vi "PromVIEW Instantiate WS.vi"(8 "error in (no error)":errorcluster, 9 "Web Resources Base Path":path, 10 "Web Service Name":string, 11 "Project Reference":refnum<vi>) -> (0 "Error Out":errorcluster)   [LabVIEW 2020]
uses:
  <resource>/Framework/Providers/ws_project_provider/common/Web Service VI Type.ctl
  <resource>/Framework/Providers/ws_project_provider/common/Web Service VI Method.ctl
  <resource>/Framework/Providers/ws_project_provider/common/Web Service VI Output Type.ctl
  <resource>/Framework/Providers/ws_project_provider/common/Web Service VI Output Format.ctl
  <resource>/Framework/Providers/ws_project_provider/common/NI Web Service Provider.lvlib
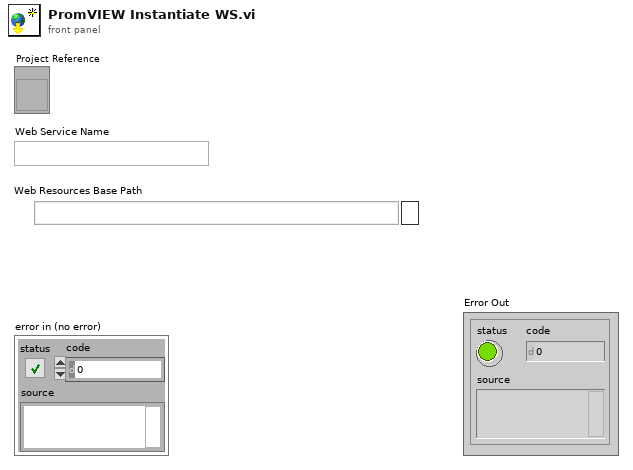
[diagram p1: front panel]
types:
  T1 = typedef "NI Web Service Provider.lvlib/Web Service VI Output Format.ctl" = enum16{"<DUMMY>", "Text", "XML", "HTML", "JSON"}
  T2 = typedef "NI Web Service Provider.lvlib/Web Service VI Output Type.ctl" = enum16{"Terminal", "Stream"}
  T3 = typedef "NI Web Service Provider.lvlib/Web Service VI Method.ctl" = enum16{"<DUMMY>", "GET", "PUT", "POST", "DELETE", "OPTIONS", "HEAD", "TRACE"}
  T4 = typedef "NI Web Service Provider.lvlib/Web Service VI Type.ctl" = enum16{"<DUMMY>", "Web Method", "Auxiliary", "Internal", "Content"}
  T5 = cluster{"Item URL":string, "Item ID":string, "Item Index":i32, "Specific Type":string}
  T6 = typedef "ItemRef.ctl" = u64
  T7 = typedef "NI Web Service Provider.lvlib/Web Service VI.ctl" = cluster{"item":u64, "item ID":string, "Web Service VI Type":T4, "Method":T3, "Load at startup":bool, "Keep in memory":bool, "Output type":T2, "Output format":T1, "Use headers":bool, "Buffered":bool, "Require API key":bool, "Permissions":string, "Standard URL":bool, "Include VI name in URL":bool, "Custom URL":string, "Required Privilege":string}
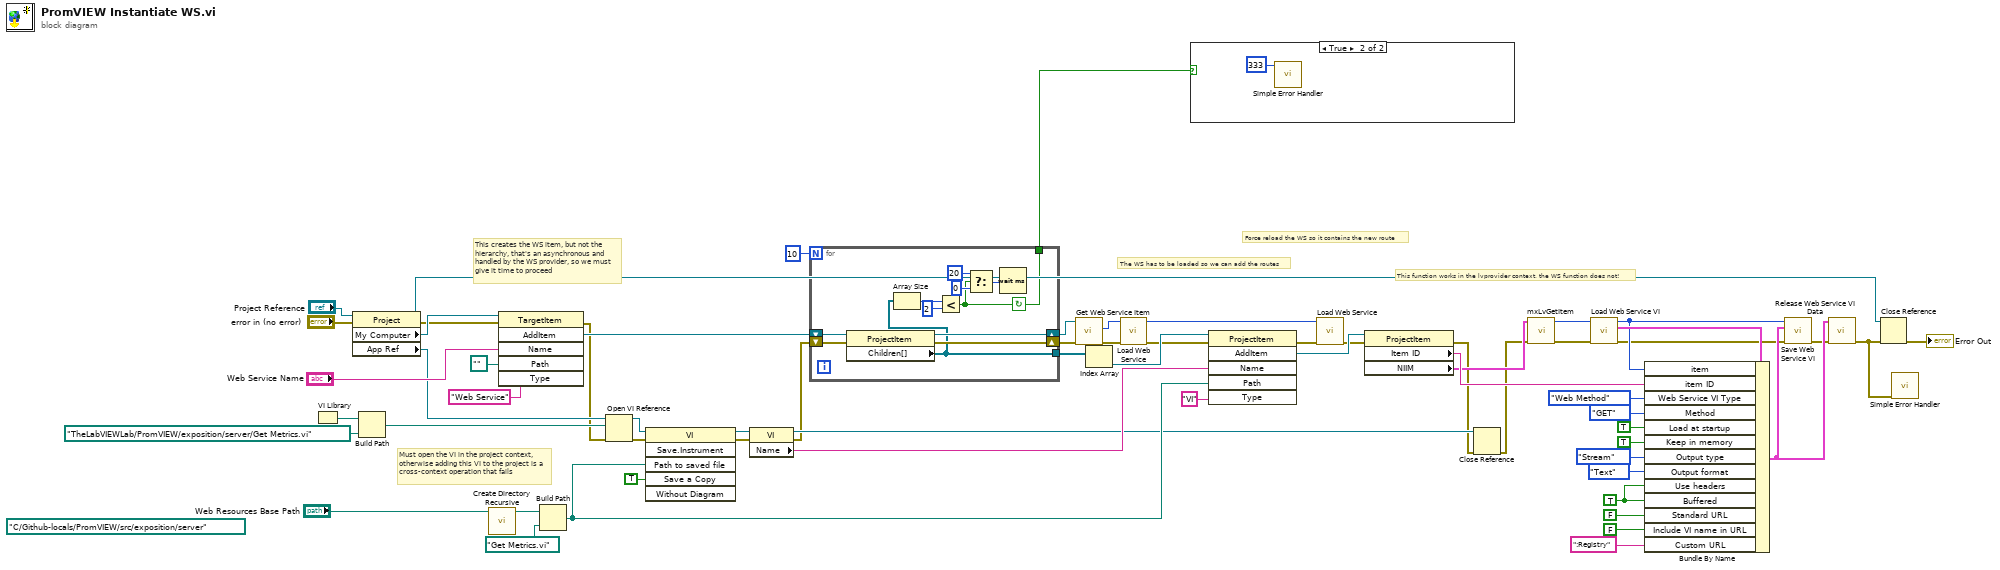
[diagram p0: block diagram]
diagram:
  w16 = TRUE ("Use headers")
  (unwired) path "C:/Github-locals/PromVIEW/src/exposition/server" ("name or relative path")
  # "Force reload the WS so it contains the new route"
  # "The WS has to be loaded so we can add the routes"
  # "This creates the WS item, but not the hierarchy, that's an asynchronous and handled by the WS provider, so we must give it time to proceed"
  # "This function works in the lvprovider context, the WS function does not!"
  # "Must open the VI in the project context, otherwise adding this VI to the project is a cross-context operation that fails"
  n1 = VI Library() -> (path=w49:path)
  n2 = property class="Project"(reference="Project Reference", error in="error in (no error)") -> (reference out=w50:refnum<vi>, error out=w56:errorcluster, "My Computer"=w62:refnum<vi>, "App Ref"=w41:refnum<vi>)
  n3 = Build Path(base path=w49, name or relative path=path "TheLabVIEWLab/PromVIEW/exposition/server/Get Metrics.vi") -> (appended path=w42:path)
  n4 = call <vilib>:"Create Directory Recursive.vi"("directory"="Web Resources Base Path") -> ("directory copy"=w58:path)  [unwired: 4 in, 2 out]
  n5 = invoke class="TargetItem" method="AddItem"(reference=w62, error in=w56, "Name"="Web Service Name", "Path"=path "", "Type"="Web Service") -> (error out=w25:errorcluster, "AddItem"=w60:refnum<vi>)  [unwired: 1 in, 4 out]
  n6 = Build Path(base path=w58, name or relative path=path "Get Metrics.vi") -> (appended path=w33:path)
  n7 = Open VI Reference(application reference (local)=w41, vi path=w42, error in (no error)=w25) -> (vi reference=w37:refnum<vi>, error out=w36:errorcluster)  [unwired: 3 in]
  n8 = invoke class="VI" method="Save.Instrument"(reference=w37, error in=w36, "Path to saved file"=w33, "Save a Copy"=TRUE) -> (reference out=w34:refnum<vi>, error out=w35:errorcluster)  [unwired: 2 in, 4 out]
  n9 = property class="VI"(reference=w34, error in=w35) -> (reference out=w31:refnum<vi>, error out=w24:errorcluster, "Name"=w46:string)
  n10 = for {
    N: 10 -> [_]
    tunnel: [w68] -> w27
    shift-right: [w73] -> w39
    shift-left: w60 -> [w74]
    shift-right: [w72] -> w30
    shift-left: w24 -> [w71]
    tunnel: [w64] -> w23
    stop <- w64 continue-if-true
    n11 = property class="ProjectItem"(reference=w74, error in=w71) -> (reference out=w73:refnum<vi>, error out=w72:errorcluster, "Children[]"=w68:refnum<vi>[])
    n12 = Array Size(array=w68) -> (size(s)=w70:i32)
    n13 = Less?(x=w70, y=2) -> (x < y?=w64:bool)
    n14 = Select(t=u32 20 ("milliseconds to wait"), s=w64, f=u32 0 ("milliseconds to wait")) -> (s? t:f=w65:u32)
    n15 = Wait (ms)(milliseconds to wait=w65) -> ()  [unwired: 1 out]
  }
  n16 = call <resource>:"Get Web Service Item.vi"("Error In"=w30, "Web service project item"=w39) -> ("Error Out"=w1:errorcluster, "Web service item"=w2:u64)  [unwired: 7 in, 1 out]
  n17 = Index Array(array=w27) -> (element=w47:refnum<vi>)  [unwired: 1 in]
  n18 = call <resource>:"Load Web Service.vi"("Error In"=w1, "Web service item"=w2) -> ("Error Out"=w40:errorcluster, "Web service item out"=w4:u64)  [unwired: 7 in, 1 out]
  n19 = case shown="True" w23 {
    frame False {
    }
    frame True {
      n20 = call <vilib>:"Simple Error Handler.vi"("error code (no error:0)"=333) -> ()  [unwired: 4 in, 5 out]
    }
  }
  n21 = invoke class="ProjectItem" method="AddItem"(reference=w47, error in=w40, "Name"=w46, "Path"=w33, "Type"="VI") -> (error out=w5:errorcluster, "AddItem"=w59:refnum<vi>)  [unwired: 1 in, 4 out]
  n22 = call <resource>:"Load Web Service.vi"("Error In"=w5, "Web service item"=w4) -> ("Error Out"=w3:errorcluster)  [unwired: 7 in, 2 out]
  n23 = property class="ProjectItem"(reference=w59, error in=w3) -> (error out=w29:errorcluster, "Item ID"=w45:string, "NIIM"=w44:T5)  [unwired: 1 out]
  n24 = Close Reference(reference=w31, error in (no error)=w29) -> (error out=w28:errorcluster)
  n25 = call <resource>:"mxLvGetItem.vi"("error in"=w28, "NIIM"=w44) -> ("error out"=w8:errorcluster, "Item"=w6:T6)  [unwired: 8 in]
  n26 = call <resource>:"Load Web Service VI.vi"("Error In"=w8, "Web service item"=w6) -> ("Error Out"=w7:errorcluster, "Web service VI"=w10:T7, "Web service item out"=w9:u64)  [unwired: 7 in]
  n27 = Bundle By Name(cluster=w10, "item"=w9, "item ID"=w45, "Web Service VI Type"=Web_Service_VI_Type."Web Method", "Method"=Web_Service_VI_Method."GET", "Load at startup"=TRUE, "Keep in memory"=TRUE, "Output type"=Web_Service_VI_Output_Type."Stream", "Output format"=Web_Service_VI_Output_Format."Text", "Use headers"=w16, "Buffered"=w16, "Standard URL"=FALSE, "Include VI name in URL"=FALSE, "Custom URL"=":Registry" ("string")) -> (w13:T7)
  n28 = call <resource>:"Save Web Service VI.vi"("Error In"=w7, "Web service VI"=w13, "Web service item"=w9) -> ("Error Out"=w12:errorcluster)  [unwired: 6 in, 2 out]
  n29 = call <resource>:"Release Web Service VI Data.vi"("Error In"=w12, "Web service VI"=w13) -> ("Error Out"=w43:errorcluster)  [unwired: 9 in]
  n30 = Close Reference(reference=w50, error in (no error)=w43) -> (error out=→"Error Out":errorcluster)
  n31 = call <vilib>:"Simple Error Handler.vi"("error in (no error)"=w43) -> ()  [unwired: 4 in, 5 out]
